vi "Zaber A Series Streaming.vi"() -> ()   [LabVIEW 2013]
doc: "Streaming lets you queue a number of commands to be completed in series. With the A-MCB2 controller it can address two and the movement of them is co-ordinated to make lines, arcs, or circles. \n\nWhen you press run this example will home, then execute each of the commands in the Stream Commands list.\n\n<b>NOTE: This example supports the A-MCB2 model only</b>"
uses:
  Zaber A Series.lvlib
panel:
  in  "VISA resource name":refnum<visa-resource-name>
  in  "Stream Commands":string[][](table)=[["stream 1 line rel 20000 20000"], ["stream 1 circle rel cw 10000 0"], ["stream 1 wait 2000"], ["stream 1 line abs 0 0"]]
  # "(c) 2014 Zaber Technologies.  ALL RIGHTS RESERVED."
  # "Streaming lets you queue a number of commands to be completed in series. With the A-MCB2 controller it can address two and the movement of them is co-ordinated to make lines, arcs, or circles. \n\nWhen you press run this example will home, then execute each of the commands in the Stream Commands list."
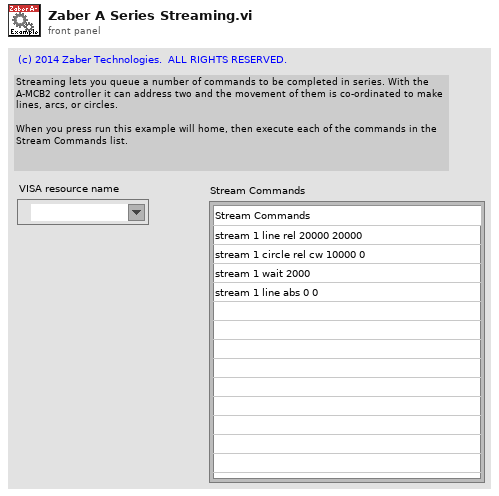
[diagram p1: front panel]
types:
  T1 = cluster{"Device":string, "Axis":string, "Reply Flag":string, "Status":string, "Warning Flags":string, "Data":string}[]
  T2 = cluster{"Device":string, "Axis":string, "Reply Flag":string, "Status":string, "Warning Flags":string, "Data":string}
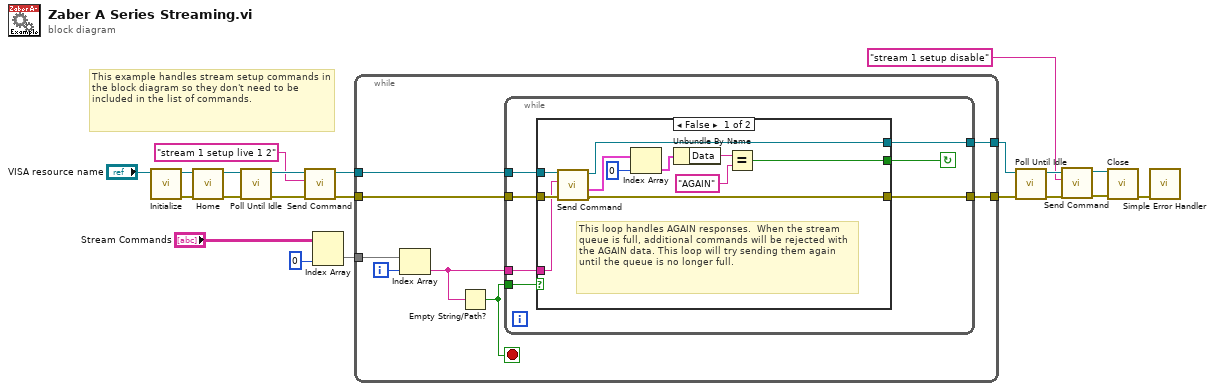
[diagram p0: block diagram]
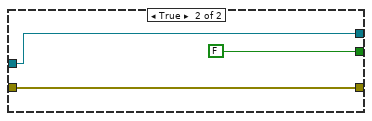
[diagram p2: hidden frame]
diagram:
  # "This example handles stream setup commands in the block diagram so they don't need to be included in the list of commands."
  n1 = call "Initialize.vi"("VISA resource name"="VISA resource name") -> ("error out"=w20:errorcluster, "VISA resource name out"=w21:refnum<visa-resource-name>)  [unwired: 9 in]
  n2 = call "Home.vi"("error in (no error)"=w20, "VISA resource name"=w21) -> ("error out"=w15:errorcluster, "VISA resource name out"=w16:refnum<visa-resource-name>)  [unwired: 8 in]
  n3 = call "Poll Until Idle.vi"("error in (no error)"=w15, "VISA resource name"=w16) -> ("error out"=w9:errorcluster, "VISA resource name out"=w10:refnum<visa-resource-name>)  [unwired: 8 in]
  n4 = call "Send Command.vi"("error in (no error)"=w9, "Command"="stream 1 setup live 1 2" ("Data"), "VISA resource name"=w10) -> ("error out"=w8:errorcluster, "VISA resource name out"=w7:refnum<visa-resource-name>)  [unwired: 4 in, 3 out]
  n5 = Index Array(array="Stream Commands", index (col)=0 ("disabled index (col)")) -> (element=w12:string[])  [unwired: 1 in]
  n6 = while {
    tunnel: [w29] -> w18
    tunnel: [w28] -> w17
    tunnel: w12 -> [w26]
    tunnel: w7 -> [w25]
    tunnel: w8 -> [w24]
    i -> [w27]
    stop <- w23 stop-if-true
    n7 = Index Array(array=w26, index=w27) -> (element=w22:string)
    n8 = Empty String/Path?(string/path=w22) -> (empty?=w23:bool)
    n9 = while {
      tunnel: [w35] -> w29
      tunnel: [w34] -> w28
      tunnel: w22 -> [w33]
      tunnel: w23 -> [w32]
      tunnel: w25 -> [w31]
      tunnel: w24 -> [w30]
      stop <- w36 continue-if-true
      n10 = case shown="False" w32 {
        tunnel: [w43 FALSE] -> w36
        tunnel: [w39 w50] -> w35
        tunnel: [w40 w49] -> w34
        tunnel: w33 -> [w37 _]
        tunnel: w31 -> [w42 w50]
        tunnel: w30 -> [w41 w49]
        frame False {
          # "This loop handles AGAIN responses.  When the stream queue is full, additional commands will be rejected with the AGAIN data. This loop will try sending them again until the queue is no longer full."
          n11 = call "Send Command.vi"("error in (no error)"=w41, "Command"=w37, "VISA resource name"=w42) -> ("error out"=w40:errorcluster, "Response Bundle Array"=w38:T1, "VISA resource name out"=w39:refnum<visa-resource-name>)  [unwired: 4 in, 2 out]
          n12 = Index Array(array=w38, index=0) -> (element=w46:T2)
          n13 = Unbundle By Name(w46) -> ("Data"=w45:string)
          n14 = Equal?(x=w45, y="AGAIN") -> (x = y?=w43:bool)
        }
        frame True {
        }
      }
    }
  }
  n15 = call "Poll Until Idle.vi"("error in (no error)"=w17, "VISA resource name"=w18) -> ("error out"=w3:errorcluster, "VISA resource name out"=w5:refnum<visa-resource-name>)  [unwired: 8 in]
  n16 = call "Send Command.vi"("error in (no error)"=w3, "Command"="stream 1 setup disable" ("Data"), "VISA resource name"=w5) -> ("error out"=w2:errorcluster, "VISA resource name out"=w4:refnum<visa-resource-name>)  [unwired: 4 in, 3 out]
  n17 = call "Close.vi"("error in (no error)"=w2, "VISA resource name"=w4) -> ("error out"=w19:errorcluster)  [unwired: 9 in]
  n18 = call <vilib>:"Simple Error Handler.vi"("error in (no error)"=w19) -> ()  [unwired: 4 in, 5 out]
